vi "MWSettings.vi"(1 "set?":bool, 2 "MW Settings":T1={"Controller ID"=4, "Interface"={"Interface"=4, "COM-Port"=0, "Baudrate"=0, "I/O-Adress (ISA)"=0}, "Stage"={"Pitch [mm/U]"={"X"=10.0, "Y"=10.0, "Z"=0.0, "A"=0.0}, "Joy Velocity [U/s]"={"X"=10.0, "Y"=10.0, "Z"=0.0, "A"=0.0}, "Acceleration [m/s²]"={"X"=10.0, "Y"=10.0, "Z"=0.0, "A"=0.0}}} {"Stage"."Acceleration [m/s²]"."A" format="%.2f"; "Stage"."Acceleration [m/s²]"."Z" format="%.2f"; "Stage"."Acceleration [m/s²]"."Y" format="%.2f"; "Stage"."Acceleration [m/s²]"."X" min=0.0 max=10.0 format="%.2f"; "Stage"."Pitch [mm/U]"."A" format="%.2f"; "Stage"."Pitch [mm/U]"."Z" format="%.2f"; "Stage"."Pitch [mm/U]"."Y" format="%.2f"; "Stage"."Pitch [mm/U]"."X" format="%.2f"; "Stage"."Joy Velocity [U/s]"."A" format="%.2f"; "Stage"."Joy Velocity [U/s]"."Z" format="%.2f"; "Stage"."Joy Velocity [U/s]"."Y" format="%.2f"; "Stage"."Joy Velocity [U/s]"."X" format="%.2f"; "Interface"."Interface" items=["", "RS232", "", "ISA", "PCI"]}) -> (0 "MW Settings out":T1={"Controller ID"=4, "Interface"={"Interface"=4, "COM-Port"=0, "Baudrate"=0, "I/O-Adress (ISA)"=0}, "Stage"={"Pitch [mm/U]"={"X"=10.0, "Y"=10.0, "Z"=0.0, "A"=0.0}, "Joy Velocity [U/s]"={"X"=10.0, "Y"=10.0, "Z"=0.0, "A"=0.0}, "Acceleration [m/s²]"={"X"=10.0, "Y"=10.0, "Z"=0.0, "A"=0.0}}} {"Stage"."Acceleration [m/s²]"."A" format="%.2f"; "Stage"."Acceleration [m/s²]"."Z" format="%.2f"; "Stage"."Acceleration [m/s²]"."Y" format="%.2f"; "Stage"."Acceleration [m/s²]"."X" min=0.0 max=10.0 format="%.2f"; "Stage"."Pitch [mm/U]"."A" format="%.2f"; "Stage"."Pitch [mm/U]"."Z" format="%.2f"; "Stage"."Pitch [mm/U]"."Y" format="%.2f"; "Stage"."Pitch [mm/U]"."X" format="%.2f"; "Stage"."Joy Velocity [U/s]"."A" format="%.2f"; "Stage"."Joy Velocity [U/s]"."Z" format="%.2f"; "Stage"."Joy Velocity [U/s]"."Y" format="%.2f"; "Stage"."Joy Velocity [U/s]"."X" format="%.2f"; "Interface"."Interface" items=["", "RS232", "", "ISA", "PCI"]})   [LabVIEW 2009]
uses:
  MW settings.ctl
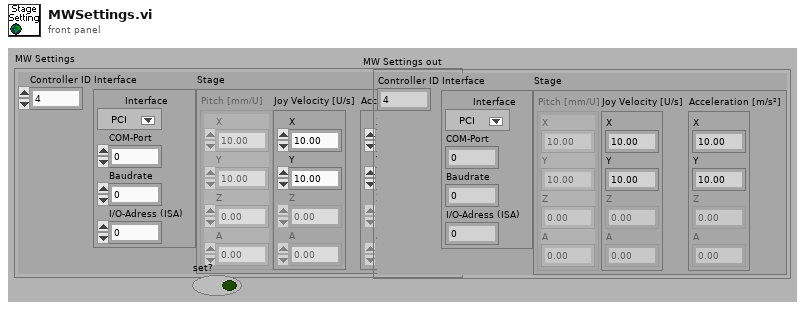
[diagram p1: front panel]
types:
  T1 = typedef "MW settings.ctl" = cluster{"Controller ID":i32, "Interface":cluster{"Interface":u32, "COM-Port":u32, "Baudrate":u32, "I/O-Adress (ISA)":u32}, "Stage":cluster{"Pitch [mm/U]":cluster{"X":dbl, "Y":dbl, "Z":dbl, "A":dbl}, "Joy Velocity [U/s]":cluster{"X":dbl, "Y":dbl, "Z":dbl, "A":dbl}, "Acceleration [m/s²]":cluster{"X":dbl, "Y":dbl, "Z":dbl, "A":dbl}}}
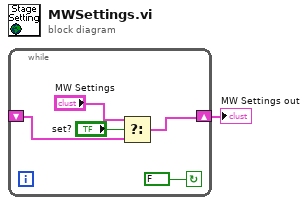
[diagram p0: block diagram]
diagram:
  n1 = while {
    shift-right: [w3] -> w1
    shift-left: _ -> [w4]
    stop <- FALSE continue-if-true
    n2 = Select(t="MW Settings", s="set?", f=w4) -> (s? t:f=w3:T1)
  }
  "MW Settings out" <- w1
